vi "Set Switch.vi"(8 "error in (no error)":errorcluster, 10 "Switch Settings":bool[](array[boolean]), 11 "4ChannelSPDTRelay in":refnum<class "4ChannelSPDTRelay.lvclass">) -> (0 "error out":errorcluster, 3 "4ChannelSPDTRelay out":refnum<class "4ChannelSPDTRelay.lvclass">)   [LabVIEW 2020, in "CTI-Peripheral.lvlib" / "4ChannelSPDTRelay.lvclass"]
uses:
  4ChannelSPDTRelay.lvclass
  4ChannelSPDTRelay.lvclass/4ChannelSPDTRelay.ctl
  CTI/I2C Connection/I2C Connection.lvclass/I2C Connection.ctl
  CTI/Session/I2C Write Data.vi
  CTI/I2C Connection/I2C Connection.lvclass
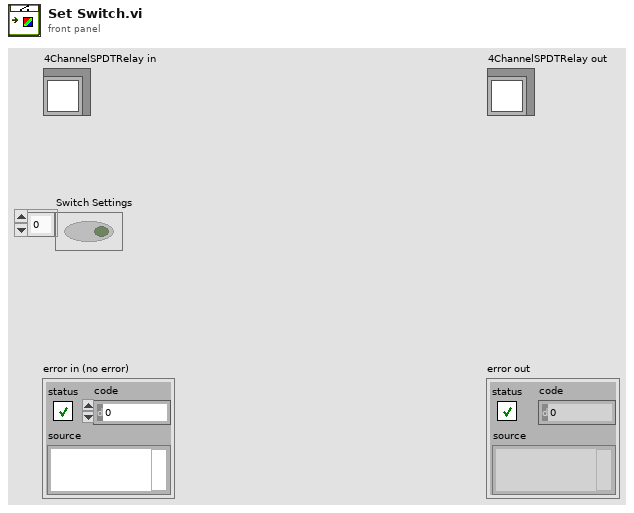
[diagram p1: front panel]
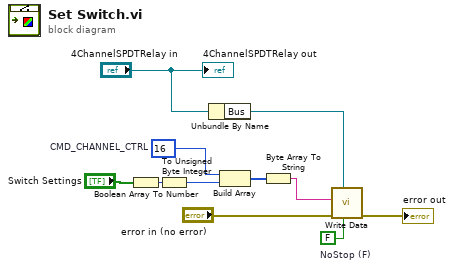
[diagram p0: block diagram]
diagram:
  w1 = u8 16  # CMD_CHANNEL_CTRL
  w7 = FALSE  # NoStop (F)
  n1 = Boolean Array To Number(Boolean array="Switch Settings") -> (number=w4:u32)
  n2 = To Unsigned Byte Integer(number=w4) -> (unsigned 8bit integer=w2:u8)
  n3 = Unbundle By Name("4ChannelSPDTRelay in") -> ("Bus"=w8:refnum<class "I2C Connection.lvclass">)
  n4 = Build Array(w1, w2) -> (w11:u8[])
  n5 = Byte Array To String(unsigned byte array=w11) -> (string=w9:string)
  n6 = call "Write Data.vi"("NoStop (F)"=w7, "I2C Connection"=w8, "error in (no error)"="error in (no error)", "Data"=w9) -> ("error out"=→"error out":errorcluster)  [unwired: 7 in]
  "4ChannelSPDTRelay out" <- "4ChannelSPDTRelay in"
